vi "plot_results.vi"(11 "IntensityGraph in":refnum<vi>) -> (1 "Intensity Graph":dbl[][](graph), 3 "Run Completed":timestamp)   [LabVIEW 2019]
uses:
  lib/libConvectionDiffusionWrapper/libConvectionDiffusionWrapper.lvlib
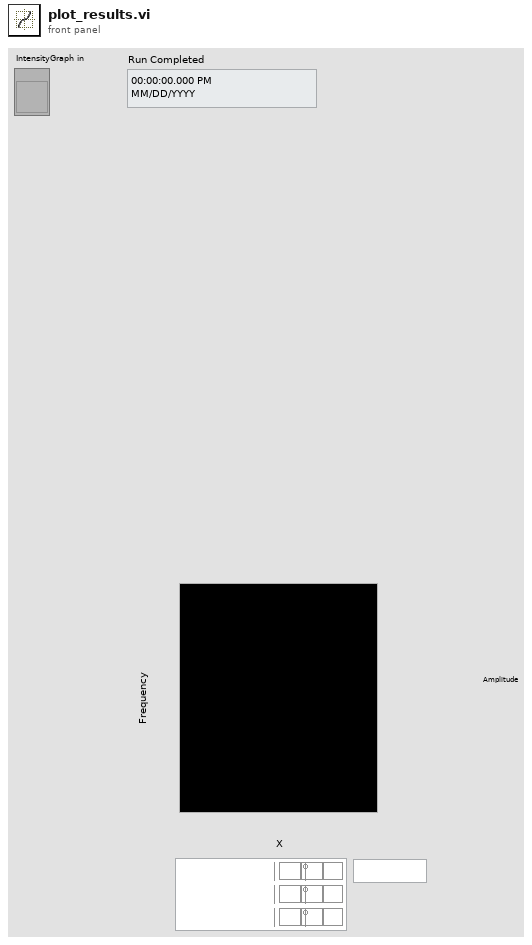
[diagram p1: front panel]
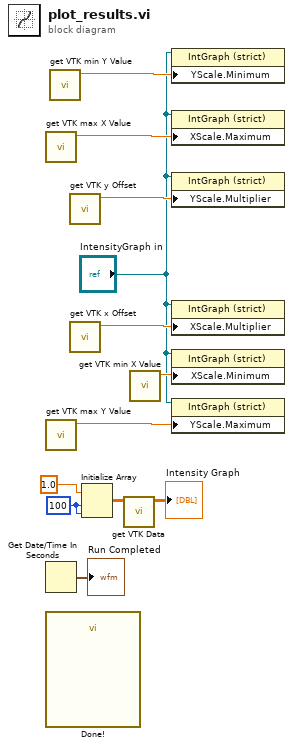
[diagram p0: block diagram]
diagram:
  w4 = 100 ("dimension size")
  n1 = call "get VTK max X Value.vi"() -> ("function return"=w7:dbl)  [unwired: 10 in, 1 out]
  n2 = call "get VTK max Y Value.vi"() -> ("function return"=w8:dbl)  [unwired: 10 in, 1 out]
  n3 = Get Date/Time In Seconds() -> (seconds since 1Jan1904=→"Run Completed":timestamp)
  n4 = call "Done!"() -> ()  [unwired: 10 in, 2 out]
  n5 = call "get VTK min Y Value.vi"() -> ("function return"=w5:dbl)  [unwired: 10 in, 1 out]
  n6 = call "get VTK y Offset.vi"() -> ("function return"=w10:dbl)  [unwired: 10 in, 1 out]
  n7 = call "get VTK x Offset.vi"() -> ("function return"=w9:dbl)  [unwired: 10 in, 1 out]
  n8 = Initialize Array(1.0 ("element"), w4, w4) -> (w11:dbl[][])
  n9 = call "get VTK Data.vi"("VTKDataIn"=w11) -> ("VTKDataOut"=→"Intensity Graph":dbl[][])  [unwired: 9 in, 1 out]
  n10 = call "get VTK min X Value.vi"() -> ("function return"=w6:dbl)  [unwired: 10 in, 1 out]
  n11 = property on="Property Node" class="IntGraph (strict)"(reference="IntensityGraph in", "YScale.Minimum"=w5) -> ()  [unwired: 1 in, 2 out]
  n12 = property on="Property Node" class="IntGraph (strict)"(reference="IntensityGraph in", "XScale.Maximum"=w7) -> ()  [unwired: 1 in, 2 out]
  n13 = property on="Property Node" class="IntGraph (strict)"(reference="IntensityGraph in", "YScale.Multiplier"=w10) -> ()  [unwired: 1 in, 2 out]
  n14 = property on="Property Node" class="IntGraph (strict)"(reference="IntensityGraph in", "XScale.Multiplier"=w9) -> ()  [unwired: 1 in, 2 out]
  n15 = property on="Property Node" class="IntGraph (strict)"(reference="IntensityGraph in", "XScale.Minimum"=w6) -> ()  [unwired: 1 in, 2 out]
  n16 = property on="Property Node" class="IntGraph (strict)"(reference="IntensityGraph in", "YScale.Maximum"=w8) -> ()  [unwired: 1 in, 2 out]
